vi "http add header to set.vi"(6 "continuation?":bool, 7 "override on duplicate?":bool, 9 "header field data":string, 10 "header field name":string, 11 "headers in":T1) -> (3 "headers out":T1)   [LabVIEW 2016, in "http headers.lvlib"]
uses:
  headers/http headers.lvlib
  http header data.ctl
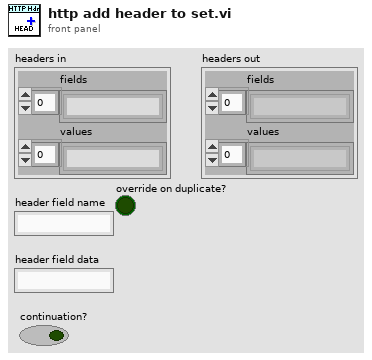
[diagram p1: front panel]
types:
  T1 = typedef "http headers.lvlib/http header data.ctl" = cluster{"fields":string[], "values":string[]}
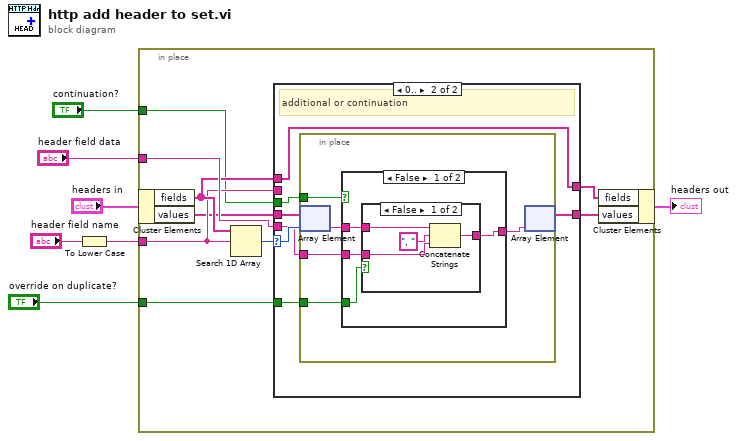
[diagram p0: block diagram]
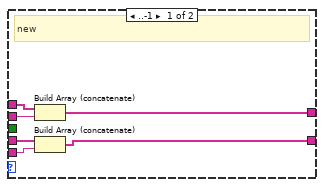
[diagram p2: hidden frame]
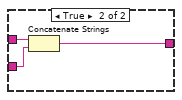
[diagram p4: hidden frame]
diagram:
  n1 = To Lower Case(string="header field name") -> (all lower case string=w1:string)
  n2 = in-place {
    in-place-border: w1 -> [w13]
    in-place-border: "header field data" -> [w16]
    in-place-border: "continuation?" -> [w9]
    in-place-border: "override on duplicate?" -> [w8]
    n3 = in-place-cluster #1("headers in") -> ("fields"=w14:string[], "values"=w11:string[])
    n4 = Search 1D Array(1D array=w14, element=w13) -> (index of element=w15:i32)  [unwired: 1 in]
    n5 = case shown="0.." w15 {
      selector: w15 -> [_ w26]
      tunnel: w16 -> [w17 w24]
      tunnel: w14 -> [w22 w29]
      tunnel: w13 -> [w21 _]
      tunnel: [w20 w29] -> w12
      tunnel: w11 -> [w19 w28]
      tunnel: [w18 w27] -> w10
      tunnel: w9 -> [_ w25]
      tunnel: w8 -> [_ w23]
      frame ..-1 {
        # "new"
        n6 = Build Array (concatenate)(w22, w21) -> (w20:string[])
        n7 = Build Array (concatenate)(w19, w17) -> (w18:string[])
      }
      frame 0.. {
        # "additional or continuation"
        n8 = in-place {
          in-place-border: w25 -> [w34]
          in-place-border: w24 -> [w32]
          in-place-border: w23 -> [w30]
          n9 = in-place-array #2(w28, w26) -> (w33:string)
          n10 = case shown="False" w34 {
            tunnel: [w37 w44] -> w31
            tunnel: w33 -> [w38 w46]
            tunnel: w32 -> [w36 w45]
            tunnel: w30 -> [w35 _]
            frame False {
              n11 = case shown="False" w35 {
                tunnel: w38 -> [w42 _]
                tunnel: [w41 w43] -> w37
                tunnel: w36 -> [w40 w43]
                frame False {
                  n12 = Concatenate Strings(w42, ", " ("string"), w40) -> (w41:string)
                }
                frame True {
                }
              }
            }
            frame True {
              n13 = Concatenate Strings(w46, w45) -> (w44:string)
            }
          }
          n14 = in-place-array #2(w31) -> (w27:string[])  [unwired: 1 out]
        }
      }
    }
    n15 = in-place-cluster #1("fields"=w12, "values"=w10) -> (→"headers out":T1)
  }
